vi "niusrprios Configure Bitfile.vi"(0 "USRP RIO device":T1, 5 "which bitfile":string(combo)="Time", 11 "error in":errorcluster) -> (4 "USRP RIO device":T1, 6 "bitfile":path, 15 "error out":errorcluster)   [LabVIEW 2015]
uses:
  <vilib>/userdefined/Silver/nirio_resource_slv.ctl
  <vilib>/regexp/Match Regular Expression.xnode
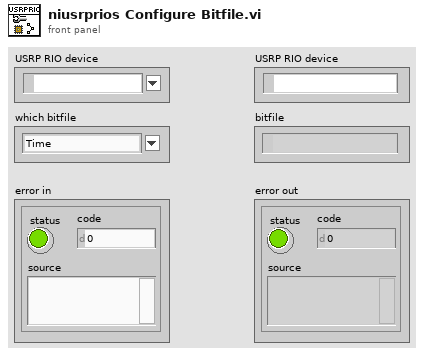
[diagram p1: front panel]
types:
  T1 = typedef "nirio_resource_slv.ctl" = tag
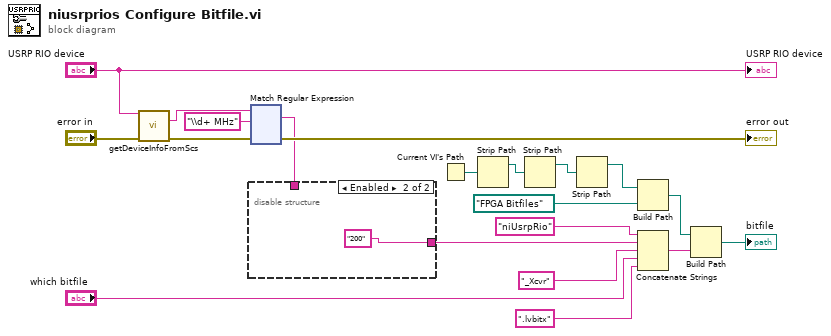
[diagram p0: block diagram]
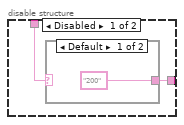
[diagram p2: hidden frame]
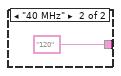
[diagram p3: hidden frame]
diagram:
  n1 = call <vilib>:"getDeviceInfoFromScs.vi"("rio device"="USRP RIO device", "error in"="error in") -> ("product name"=w4:string, "error out"=w5:errorcluster)  [unwired: 9 in, 3 out]
  n2 = xnode "Match Regular Expression"("input string"=w4, "regular expression"="\\d+ MHz", "error in"=w5) -> ("whole match"=w2:string, "error out"=→"error out":errorcluster)  [unwired: 3 in, 3 out]
  n3 = disable-structure shown="Enabled" {
    disable-tunnel: w2 -> [w22 _]
    disable-tunnel: [w21 "200" ("format string")] -> w1
    frame Disabled {
      n4 = case shown="Default" w22 {
        tunnel: ["200" ("format string") "120" ("format string")] -> w21
        frame Default {
        }
        frame "40 MHz" {
        }
      }
    }
    frame Enabled {
    }
  }
  n5 = Current VI's Path() -> (path=w20:path)
  n6 = Strip Path(path=w20) -> (stripped path=w17:path)  [unwired: 1 out]
  n7 = Strip Path(path=w17) -> (stripped path=w16:path)  [unwired: 1 out]
  n8 = Strip Path(path=w16) -> (stripped path=w15:path)  [unwired: 1 out]
  n9 = Build Path(base path=w15, name or relative path=path "FPGA Bitfiles") -> (appended path=w18:path)
  n10 = Concatenate Strings("niUsrpRio" ("format string"), w1, "_Xcvr" ("format string"), "which bitfile", ".lvbitx" ("format string")) -> (w11:string)
  n11 = Build Path(base path=w18, name or relative path=w11) -> (appended path=→"bitfile":path)
  "USRP RIO device" <- "USRP RIO device"
